vi "Potting Data - BBM Pad Groups.vi"(8 "error in":errorcluster, 9 "Config Manager":refnum<class "Config Manager Class.lvclass">, 10 "Potting Selection BBM Bond Pads":bool[](array[boolean]), 11 "BBM Bond Pad References":T2[](array[typedef])) -> (0 "error out":errorcluster, 3 "Potting Lines":T1[](array[typedef]))   [LabVIEW 2011]
uses:
  Shared Components/Utils/Type Definitions/Fiducial Image.ctl
  Shared Components/Vec3d Class/Vec3d Class.lvclass
  Shared Components/Utils/Type Definitions/Physical Image.ctl
  <vilib>/vision/Image Controls.llb/IMAQ Image.ctl
  Shared Components/Utils/Type Definitions/Fiducial with Source.ctl
  Shared Components/Config Manager Class/Config Manager Class.lvclass
  Shared Components/Utils/Type Definitions/3d Line.ctl
  Shared Components/Config Manager Class/Type Definitions/Part Type.ctl
  Shared Components/Config Manager Class/Read Geometry Definition Integer.vi
  Shared Components/Config Manager Class/Read Geometry Definition Double.vi
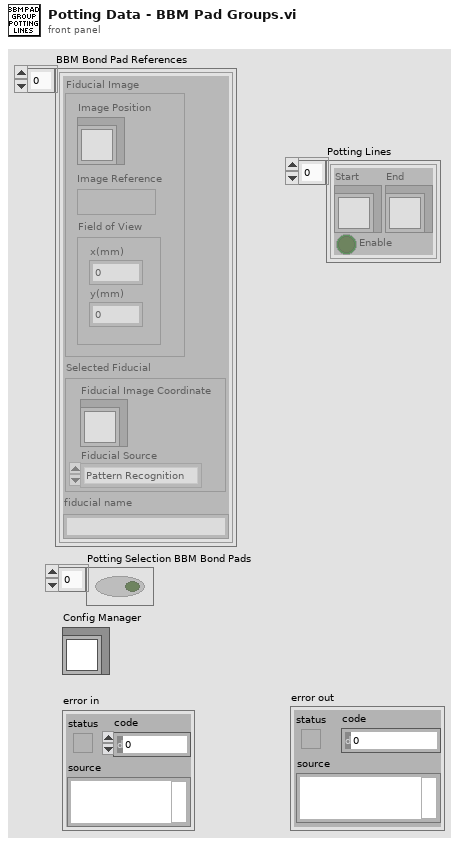
[diagram p1: front panel]
types:
  T1 = typedef "3d Line.ctl" = cluster{"Start":refnum<class "Vec3d Class.lvclass">, "End":refnum<class "Vec3d Class.lvclass">, "Enable":bool}
  T2 = typedef "Fiducial Image.ctl" = cluster{"Fiducial Image":T3, "Selected Fiducial":T5, "fiducial name":string}
  T3 = typedef "Physical Image.ctl" = cluster{"Image Position":refnum<class "Vec3d Class.lvclass">, "Image Reference":T4, "Field of View":cluster{"x(mm)":dbl, "y(mm)":dbl}}
  T4 = typedef "IMAQ Image.ctl" = refnum<image>
  T5 = typedef "Fiducial with Source.ctl" = cluster{"Fiducial Image Coordinate":refnum<class "Vec3d Class.lvclass">, "Fiducial Source":enum16{"Pattern Recognition", "User", "Error", "Default"}}
  T6 = typedef "Part Type.ctl" = enum16{"BBM", "HDI", "GLUERESERVOIR", "STAMP", "WEIGHT"}
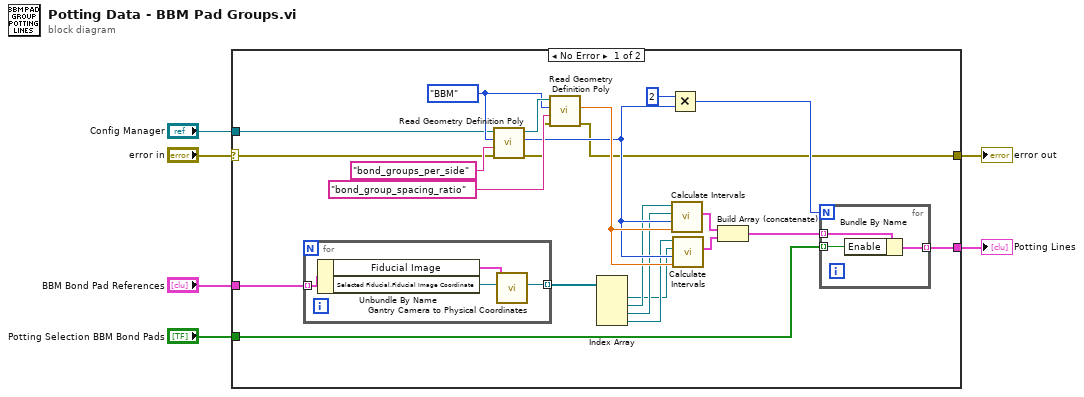
[diagram p0: block diagram]
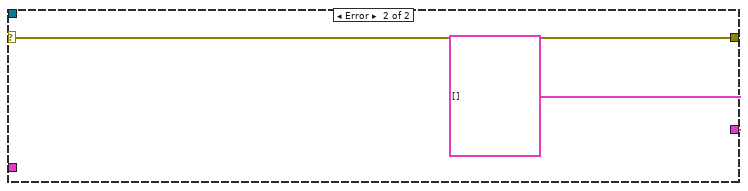
[diagram p2: hidden frame]
diagram:
  n1 = case shown="No Error" "error in" {
    selector: "error in" -> [w14 w38]
    tunnel: "Config Manager" -> [w25 _]
    tunnel: "BBM Bond Pad References" -> [w24 _]
    tunnel: "Potting Selection BBM Bond Pads" -> [w18 _]
    tunnel: [w7 T1[] [] ("appended array")] -> w2
    tunnel: [w12 w38] -> w1
    frame No Error {
      w28 = Part_Type."BBM" ("Part Type")
      n2 = for {
        tunnel: w24 -> [w36] mode=indexing
        tunnel: [w33] -> w23 mode=indexing
        n3 = Unbundle By Name(w36) -> ("Fiducial Image"=w35:T3, "Selected Fiducial.Fiducial Image Coordinate"=w34:refnum<class "Vec3d Class.lvclass">)
        n4 = call "Gantry Camera to Physical Coordinates.vi"("Image Coordinate"=w34, "Physical Image"=w35) -> ("Global Coordinate"=w33:refnum<class "Vec3d Class.lvclass">)  [unwired: 7 in, 2 out]
      }
      n5 = call-poly "Read Geometry Definition Poly.vi"("error in"=w14, "Feature"="bond_groups_per_side", "Part Type"=w28, "Config Manager in"=w25) -> ("error out"=w13:errorcluster, "Geometry Definition"=w17:i32, "Config Manager out"=w29:refnum<class "Config Manager Class.lvclass">)  [unwired: 5 in]
      n6 = call-poly "Read Geometry Definition Poly.vi"("error in"=w13, "Feature"="bond_group_spacing_ratio", "Part Type"=w28, "Config Manager in"=w29) -> ("error out"=w12:errorcluster, "Geometry Definition"=w22:dbl)  [unwired: 5 in, 1 out]
      n7 = Index Array(array=w23) -> (element #1=w8:refnum<class "Vec3d Class.lvclass">, element #2=w10:refnum<class "Vec3d Class.lvclass">, element #3=w11:refnum<class "Vec3d Class.lvclass">, element #4=w9:refnum<class "Vec3d Class.lvclass">)  [unwired: 4 in]
      n8 = Multiply(x=2, y=w17) -> (x*y=w15:i32)
      n9 = call "Calculate Intervals.vi"("gap/group ratio"=w22, "Num Intervals"=w17, "End"=w11, "Start"=w10) -> ("Intervals"=w21:T1[])  [unwired: 7 in]
      n10 = call "Calculate Intervals.vi"("gap/group ratio"=w22, "Num Intervals"=w17, "End"=w8, "Start"=w9) -> ("Intervals"=w20:T1[])  [unwired: 7 in]
      n11 = Build Array (concatenate)(w21, w20) -> (w19:T1[])
      n12 = for {
        N: w15 -> [_]
        tunnel: w19 -> [w32] mode=indexing
        tunnel: w18 -> [w31] mode=indexing
        tunnel: [w30] -> w7 mode=indexing
        n13 = Bundle By Name(cluster=w32, "Enable"=w31) -> (w30:T1)
      }
    }
    frame Error {
    }
  }
  "Potting Lines" <- w2
  "error out" <- w1
